vi "checknull.vi"(0 "error in (no error)":errorcluster, 3 "ptr":u32, 4 "error code":i32=6003) -> (2 "error out":errorcluster)   [LabVIEW 2010, in "lib1299.lvlib"]
uses:
  lib1299.lvlib
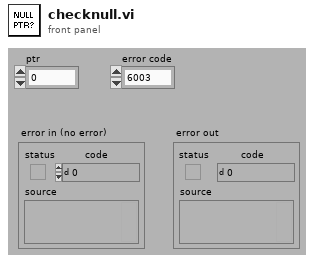
[diagram p1: front panel]
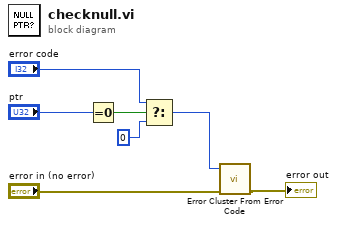
[diagram p0: block diagram]
diagram:
  n1 = Equal To 0?(x="ptr") -> (x = 0?=w6:bool)
  n2 = Select(t="error code", s=w6, f=0) -> (s? t:f=w1:i32)
  n3 = call <vilib>:"Error Cluster From Error Code.vi"("error in (no error)"="error in (no error)", "error code (0)"=w1) -> ("error out"=→"error out":errorcluster)  [unwired: 7 in]
